vi "FABR-Check Status.vi"(0 "Runtime in":T2, 2 "queue":refnum<queue>, 7 "SCL in":cluster{T1[]}[](array[cluster]), 9 "Finished":bool, 11 "error in (no error)":errorcluster) -> (4 "Runtime out":T2, 8 "SCL thru":cluster{T1[]}[](array[cluster]), 10 "stop":bool, 15 "error out":errorcluster)   [LabVIEW 2020]
uses:
  Typedefs/FABR-Runtime Data.ctl
  Typedefs/FABR-Stimulus Ticket.ctl
  Typedefs/FABR-Order.ctl
  Typedefs/FABR-Stimulus Condition.ctl
  Typedefs/FABR-Queue Data.ctl
  Typedefs/FABR-Parameters.ctl
  Typedefs/FABR-Stimulus.ctl
  Typedefs/FABR-Sequence.ctl
  Typedefs/FABR-Response.ctl
  Threshold Estimation VIs/ABR3-Threshold Estimation Parameters.ctl
  epl-vi-lib/PXI DAQ VIs/AODO/Typedefs/AODO-Action.ctl
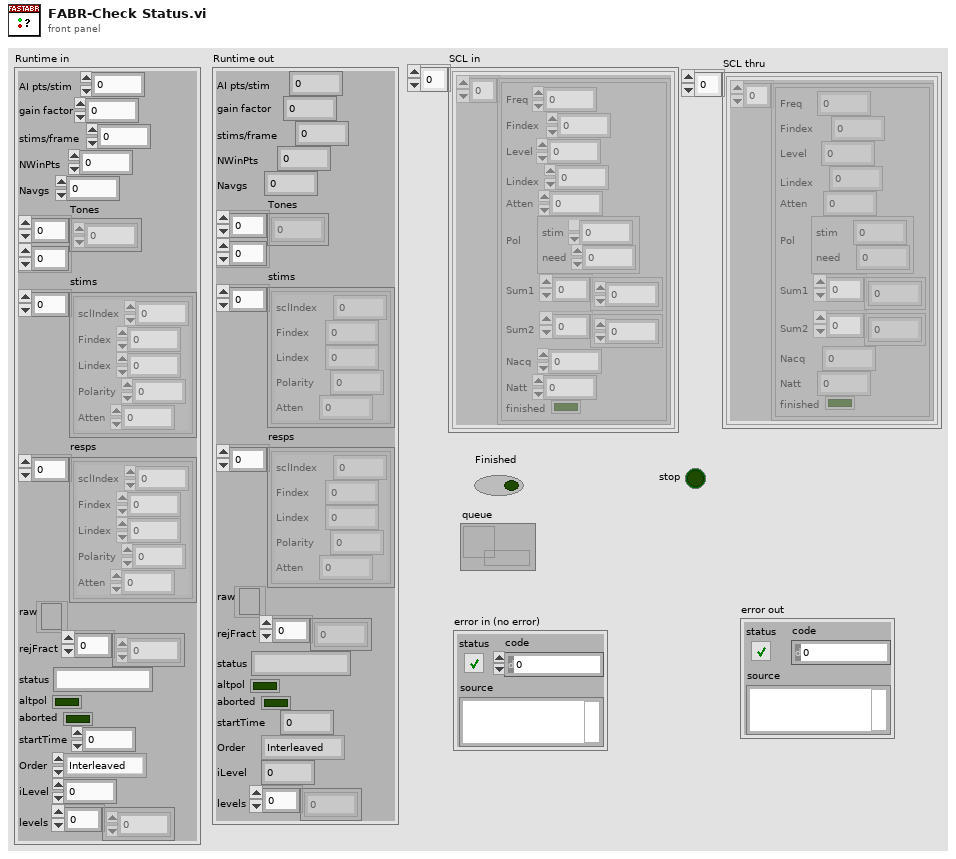
[diagram p1: front panel]
types:
  T1 = typedef "FABR-Stimulus Condition.ctl" = cluster{"Freq":dbl, "Findex":i32, "Level":dbl, "Lindex":i32, "Atten":dbl, "Pol":cluster{"stim":i32, "need":i32}, "Sum1":dbl[], "Sum2":dbl[], "Nacq":i32, "Natt":i32, "finished":bool}
  T2 = typedef "FABR-Runtime Data.ctl" = cluster{"AI pts/stim":i32, "gain factor":dbl, "stims/frame":i32, "NWinPts":i32, "Navgs":i32, "Tones":dbl[][], "stims":T3[], "resps":T3[], "raw":refnum<file>, "rejFract":dbl[], "status":string, "altpol":bool, "aborted":bool, "startTime":dbl, "Order":T4, "iLevel":i32, "levels":dbl[]}
  T3 = typedef "FABR-Stimulus Ticket.ctl" = cluster{"sclIndex":i32, "Findex":i32, "Lindex":i32, "Polarity":i32, "Atten":dbl}
  T4 = typedef "FABR-Order.ctl" = enum16{"Interleaved", "Stepped level"}
  T5 = typedef "AODO-Action.ctl" = enum16{"Configure", "Initialize", "Start", "Write", "Clean up", "Init & Start", "Config & Test", "Position", "Set AO Gains", "Zero", "Prime", "Status"}
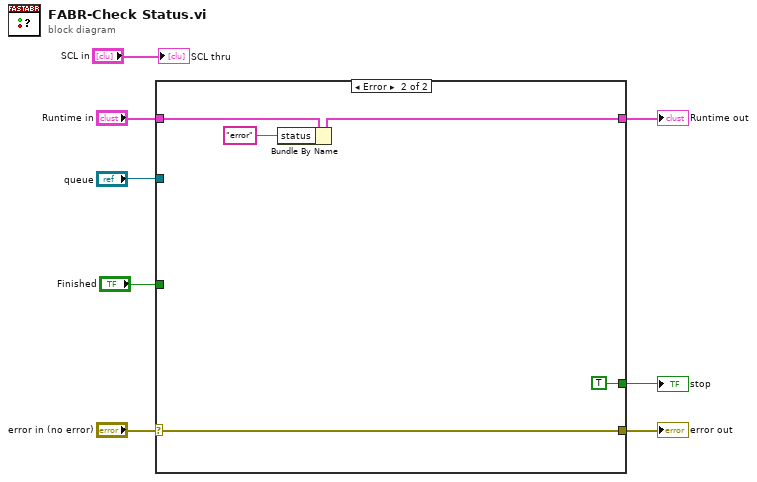
[diagram p0: block diagram]
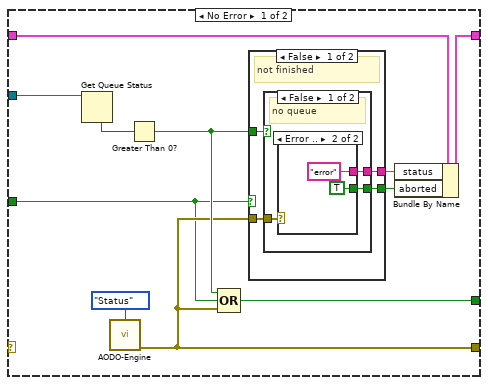
[diagram p2: hidden frame]
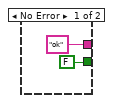
[diagram p3: hidden frame]
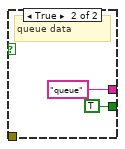
[diagram p4: hidden frame]
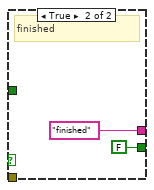
[diagram p5: hidden frame]
diagram:
  n1 = case shown="Error" "error in (no error)" {
    selector: "error in (no error)" -> [_ w39]
    tunnel: [w12 w39] -> w7
    tunnel: [w18 TRUE] -> w6
    tunnel: "queue" -> [w17 _]
    tunnel: "Runtime in" -> [w10 w37]
    tunnel: [w15 w36] -> w3
    tunnel: "Finished" -> [w9 _]
    frame No Error {
      n2 = Get Queue Status(queue=w17) -> (# elements in queue=w16:i32)  [unwired: 2 in, 7 out]
      n3 = call "AODO-Engine.vi"("Action"=AODO-Action."Status") -> ("error out"=w12:errorcluster)  [unwired: 9 in, 5 out]
      n4 = Greater Than 0?(x=w16) -> (x > 0?=w13:bool)
      n5 = Compound Arithmetic op=OR(w13, w9, w12) -> (w18:bool)
      n6 = case shown="False" w9 {
        tunnel: [w22 "finished"] -> w14
        tunnel: w13 -> [w23 _]
        tunnel: w12 -> [w21 _]
        tunnel: [w20 FALSE] -> w11
        frame False {
          # "not finished"
          n7 = case shown="False" w23 {
            tunnel: [w25 "queue"] -> w22
            tunnel: w21 -> [w26 _]
            tunnel: [w24 TRUE] -> w20
            frame False {
              # "no queue"
              n8 = case shown="Error .." w26 {
                tunnel: ["ok" "error"] -> w25
                tunnel: [FALSE TRUE] -> w24
                frame No Error {
                }
                frame Error {
                }
              }
            }
            frame True {
              # "queue data"
            }
          }
        }
        frame True {
          # "finished"
        }
      }
      n9 = Bundle By Name(cluster=w10, "status"=w14, "aborted"=w11) -> (w15:T2)
    }
    frame Error {
      n10 = Bundle By Name(cluster=w37, "status"="error") -> (w36:T2)
    }
  }
  "stop" <- w6
  "error out" <- w7
  "Runtime out" <- w3
  "SCL thru" <- "SCL in"
